vi "Instantiate.vi"(11 "error in":errorcluster) -> (4 "function manager":refnum<class "function manager.lvclass">, 15 "error out":errorcluster)   [LabVIEW 2016, in "function manager.lvclass"]
uses:
  function manager.lvclass
  functionsbase/functionbase.lvclass
  function manager.lvclass/function manager.ctl
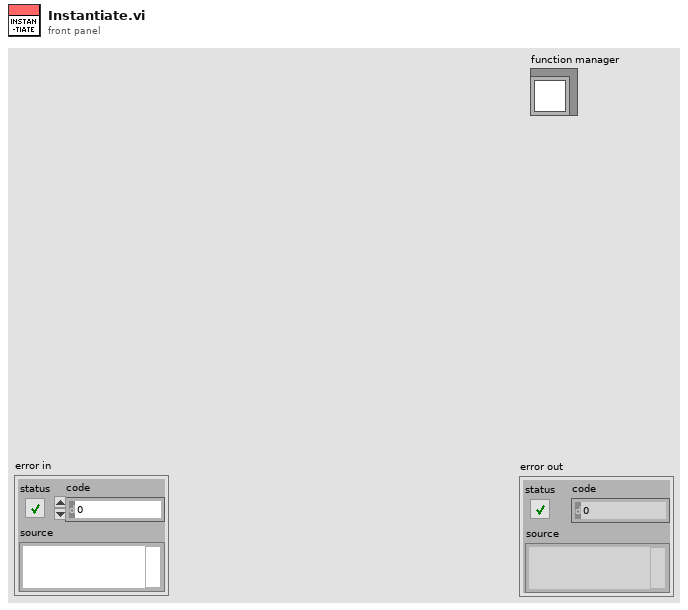
[diagram p1: front panel]
types:
  T1 = typedef "Syntax Format.ctl" = cluster{"Syntax":string, "Variable#":T2}
  T2 = typedef "Variable#.ctl" = enum16{"Zero", "One", "Two", "Three", "Four", "Five"}
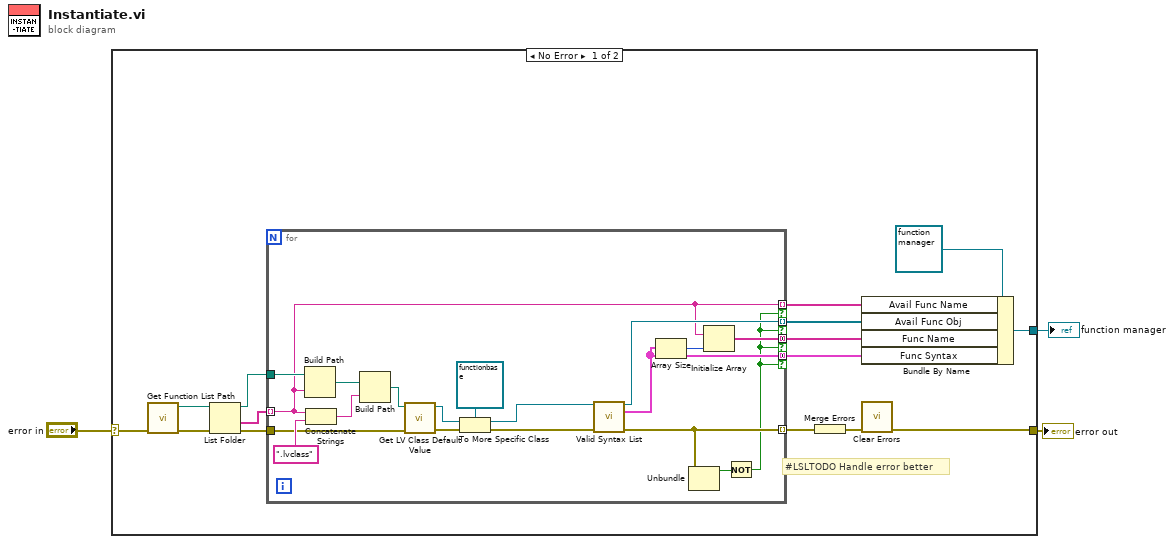
[diagram p0: block diagram]
diagram:
  n1 = case shown="No Error" "error in" {
    selector: "error in" -> [w18 w38]
    tunnel: [w10 w38] -> w2
    tunnel: [w6 _] -> w1
    frame No Error {
      # "#LSLTODO Handle error better"
      n2 = call "Get Function List Path.vi"("error in"=w18) -> ("error out"=w17:errorcluster, "Functions List Path"=w16:path)  [unwired: 9 in]
      n3 = List Folder(path=w16, error in=w17) -> (path out=w13:path, folder names=w14:string[], error out=w15:errorcluster)  [unwired: 2 in, 1 out]
      n4 = for {
        tunnel: w15 -> [w32]
        tunnel: w14 -> [w21] mode=indexing
        tunnel: w13 -> [w37]
        tunnel: [w26] -> w12 mode=indexing
        tunnel: [w24] -> w7 mode=indexing if=w19
        tunnel: [w21] -> w8 mode=indexing if=w19
        tunnel: [w23] -> w4 mode=concatenating if=w19
        tunnel: [w20] -> w5 mode=concatenating if=w19
        n5 = Build Path(base path=w37, name or relative path=w21) -> (appended path=w36:path)
        n6 = Concatenate Strings(w21, ".lvclass" ("string")) -> (w34:string)
        n7 = Build Path(base path=w36, name or relative path=w34) -> (appended path=w33:path)
        n8 = call <vilib>:"Get LV Class Default Value.vi"("error in (no error)"=w32, "class path"=w33) -> ("error out"=w31:errorcluster, "object"=w30:refnum<class>)  [unwired: 8 in]
        n9 = To More Specific Class(target class=refnum<class "functionbase.lvclass"> refnum ("functionbase.lvclass"), reference=w30, error in=w31) -> (specific class reference=w25:refnum<class "functionbase.lvclass">, error out=w27:errorcluster)
        n10 = call-dynamic "Valid Syntax List.vi"("functionbase in"=w25, "error in (no error)"=w27) -> ("functionbase out"=w24:refnum<class "functionbase.lvclass">, "Syntax List"=w23:T1[], "error out"=w26:errorcluster)  [unwired: 11 in]
        n11 = Array Size(array=w23) -> (size(s)=w22:i32)
        n12 = Unbundle(w26) -> ("status"=w28:bool)  [unwired: 2 out]
        n13 = Initialize Array(w21, w22) -> (w20:string[])
        n14 = Not(x=w28) -> (.not. x?=w19:bool)
      }
      n15 = Merge Errors(w12) -> (w11:errorcluster)
      n16 = Bundle By Name(cluster=refnum<class "function manager.lvclass"> refnum ("function manager.lvlib:function manager.lvclass"), "Avail Func Name"=w8, "Avail Func Obj"=w7, "Func Name"=w5, "Func Syntax"=w4) -> (w6:refnum<class "function manager.lvclass">)
      n17 = call <vilib>:"Clear Errors.vi"("error in (no error)"=w11) -> ("error out"=w10:errorcluster)  [unwired: 5 in, 1 out]
    }
    frame Error {
    }
  }
  "error out" <- w2
  "function manager" <- w1
